vi "Init.vi"(8 "Error In":errorcluster) -> (0 "Error Out":errorcluster, 3 "Not connected":bool)   [LabVIEW 2018]
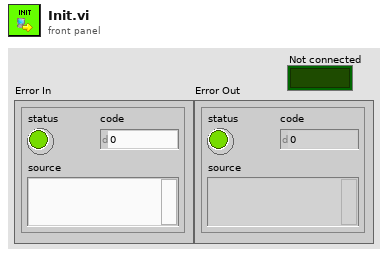
[diagram p1: front panel]
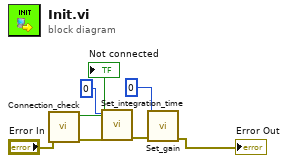
[diagram p0: block diagram]
diagram:
  n1 = call "Connection_check.vi"("error in"="Error In") -> ("error out"=w5:errorcluster, "Not connected"=→"Not connected":bool)  [unwired: 9 in]
  n2 = call "Set_integration_time.vi"("error in"=w5, "Integration Time"=u8 0) -> ("error out"=w4:errorcluster)  [unwired: 9 in]
  n3 = call "Set_gain.vi"("error in"=w4, "Gain"=u8 0) -> ("error out"=→"Error Out":errorcluster)  [unwired: 9 in]
